vi "test.vi"() -> ()   [LabVIEW 2020]
uses:
  <vilib>/addons/control/pid/pid.llb/PID (DBL).vi
  <vilib>/addons/control/pid/NI_PID_pid.lvlib
panel:
  out "双精度浮点数":dbl
  in  "SP：":dbl(slide)=43.790849673202615 min=0.0 max=0.0 scale=0.0..100.0
  in  "停止 2":bool
  out "过程变量和设定值":cluster{"initial PV":dbl, "SP:":dbl}(graph)
  in  "PID增益":T1={"比例增益(Kc)"=20.0, "积分时间（Ti，分）"=0.008, "微分时间（Td，分）"=0.001} {"微分时间（Td，分）" format="%.3f"; "积分时间（Ti，分）" format="%.3f"; "比例增益(Kc)" format="%.3f"}
  out "PV：":dbl(slide)=60.754431603254424 scale=0.0..100.0
  out "MV：":dbl(slide)=18.78965245852964 scale=-100.0..100.0
  out "操作变量":dbl(graph)
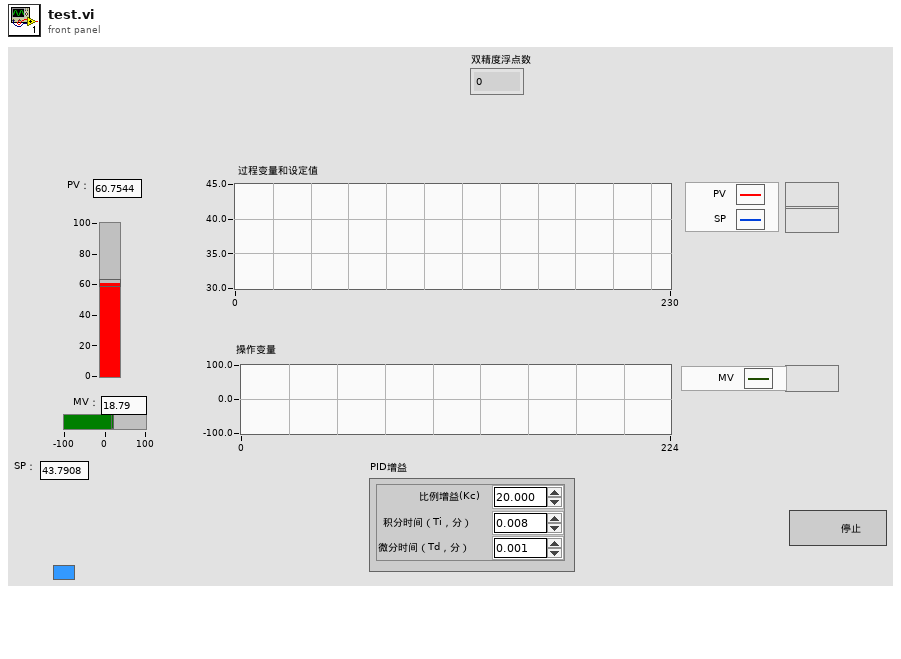
[diagram p1: front panel]
types:
  T1 = cluster{"比例增益(Kc)":dbl, "积分时间（Ti，分）":dbl, "微分时间（Td，分）":dbl}
  T2 = enum16{"open", "replace", "create", "open or create", "replace or create", "replace or create with confirmation"}
  T3 = cluster{"static gain":dbl, "lag (min)":dbl, "dead cycles":dbl, "load %":dbl, "deadband":dbl, "noise level %":dbl, "initial PV":dbl, "initial PV 2":dbl}
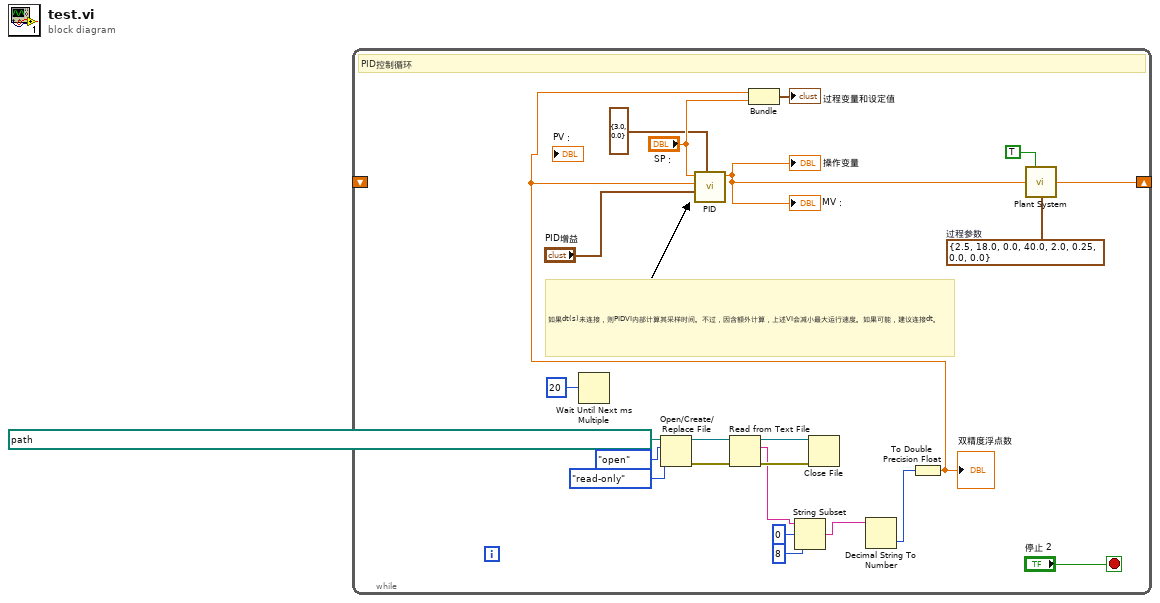
[diagram p0: block diagram]
diagram:
  n1 = while {
    shift-left: _ -> [_]
    shift-right: [w22] -> _
    stop <- "停止 2" stop-if-true
    w17 = T3 {"static gain"=2.5, "lag (min)"=18.0, "dead cycles"=0.0, "load %"=40.0, "deadband"=2.0, "noise level %"=0.25, "initial PV"=0.0, "initial PV 2"=0.0}  # 过程参数
    # "如果dt(s)未连接，则PIDVI内部计算其采样时间。不过，因含额外计算，上述VI会减小最大运行速度。如果可能，建议连接dt。"
    # "PID控制循环"
    n2 = Wait Until Next ms Multiple(millisecond multiple=u32 20 ("unsigned 32bit integer")) -> ()  [unwired: 1 out]
    n3 = Open/Create/Replace File(file path (use dialog)=path "C:/Users/20219/Desktop/project/old/A315Demo 8.8/A315Demo 7.31/A315Demo-7.30/A35Demo/bin/温度.txt" ("文件路径（使用对话框）"), operation (0:open)=T2."open" ("操作(0:open)"), access (0:read/write)=enum16{"read/write", "read-only", "write-only"}."read-only" ("权限(0:read/write)")) -> (refnum out=w12:refnum<file>, error out=w14:errorcluster)  [unwired: 3 in, 1 out]
    n4 = Read from Text File(file (use dialog)=w12, error in=w14) -> (refnum out=w13:refnum<file>, text=w6:string, error out=w15:errorcluster)  [unwired: 2 in, 1 out]
    n5 = String Subset(string=w6, offset (0)=0 ("偏移量(0)"), length (rest)=8 ("长度（剩余）")) -> (substring=w3:string)
    n6 = Close File(refnum=w13, error in=w15) -> ()  [unwired: 2 out]
    n7 = Decimal String To Number(string=w3) -> (number=w2:i32)  [unwired: 2 in, 1 out]
    n8 = To Double Precision Float(number=w2) -> (double precision float=w4:dbl)
    "双精度浮点数" <- w4
    n9 = call-poly <vilib>:"PID.vi"("output range"=cluster{"output high":dbl, "output low":dbl} {"output high"=3.0, "output low"=0.0}, "PID gains"="PID增益", "process variable"=w4, "setpoint"="SP：") -> ("output"=w18:dbl)  [unwired: 6 in, 1 out]
    "MV：" <- w18
    "操作变量" <- w18
    n10 = Bundle(w4, "SP："="SP：") -> (→"过程变量和设定值":cluster{dbl, "SP：":dbl})  [unwired: 1 in]
    n11 = call "Plant System.vi"("积分器？"=TRUE ("Integrator ?"), "设备输入"=w18, "过程参数"=w17) -> ("设备输出"=w22:dbl)  [unwired: 12 in]
  }
